vi "Parse.vi"(8 "Error In":errorcluster, 11 "object in":refnum<class "2021_11.lvclass">) -> (0 "Error Out":errorcluster, 3 "object out":refnum<class "2021_11.lvclass">)   [LabVIEW 2020, in "2021_11.lvclass"]
uses:
  2021_11.lvclass
  2021_11.lvclass/2021_11.ctl
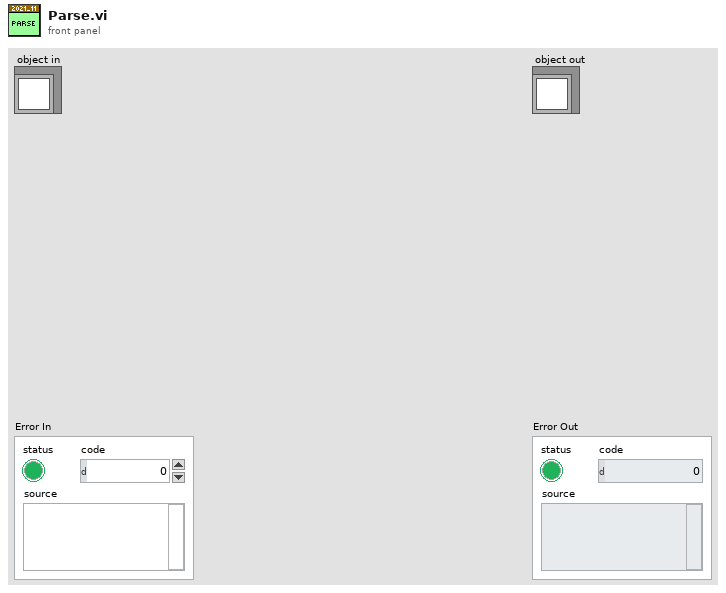
[diagram p1: front panel]
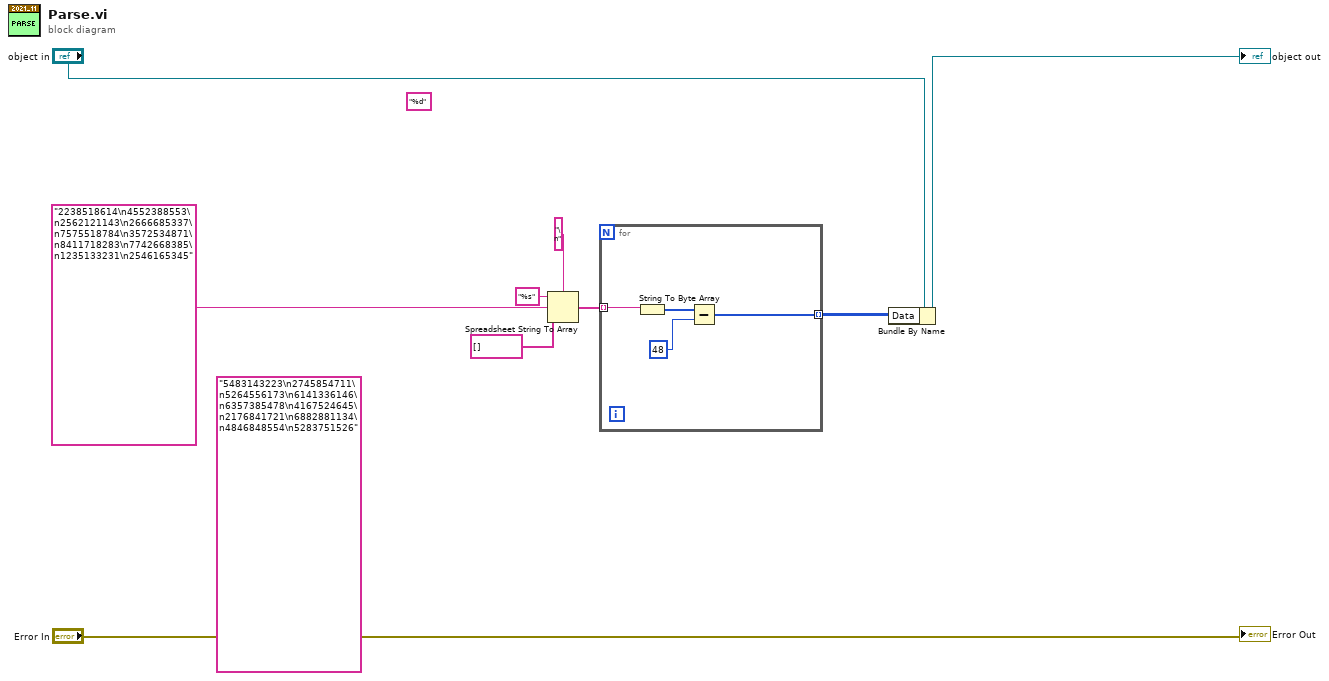
[diagram p0: block diagram]
diagram:
  (unwired) "5483143223\n2745854711\n5264556173\n6141336146\n6357385478\n4167524645\n2176841721\n6882881134\n4846848554\n5283751526" ("PuzzleInput")
  (unwired) "%d" ("format string")
  n1 = Spreadsheet String To Array(delimiter (Tab)="\n", format string="%s", spreadsheet string="2238518614\n4552388553\n2562121143\n2666685337\n7575518784\n3572534871\n8411718283\n7742668385\n1235133231\n2546165345" ("PuzzleInput"), array type (2D Dbl)=string[] []) -> (array=w3:string[])
  n2 = for {
    tunnel: w3 -> [w13] mode=indexing
    tunnel: [w10] -> w2 mode=indexing
    n3 = String To Byte Array(string=w13) -> (unsigned byte array=w12:u8[])
    n4 = Subtract(x=w12, y=48) -> (x-y=w10:i32[])
  }
  n5 = Bundle By Name(cluster="object in", "Data"=w2) -> (→"object out":refnum<class "2021_11.lvclass">)
  "Error Out" <- "Error In"
